vi "Axis_traversed.vi"(4 "Position array":sgl[][](array[numeric]) format="%.2f") -> (1 "Axis Traversed":enum16{"X traverse", "Y traverse", "Z traverse"}(ring))   [LabVIEW 2020]
uses:
  Globals/Trav_pos_global.vi
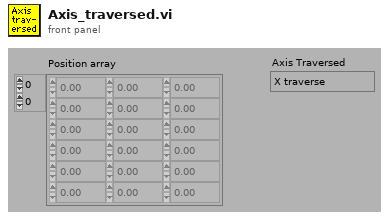
[diagram p1: front panel]
types:
  T1 = enum16{"X traverse", "Y traverse", "Z traverse"}[]
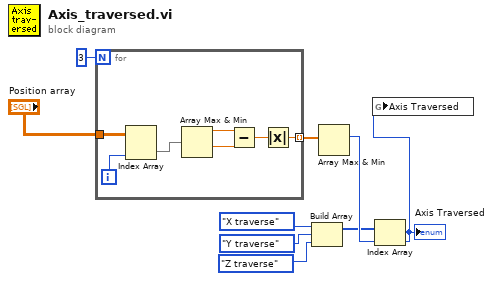
[diagram p0: block diagram]
diagram:
  n1 = for {
    N: 3 -> [_]
    tunnel: "Position array" -> [w15]
    tunnel: [w10] -> w4 mode=indexing
    i -> [w16]
    n2 = Index Array(array=w15, index (col)=w16) -> (element=w14:sgl[])  [unwired: 1 in]
    n3 = Array Max & Min(array=w14) -> (max value=w13:sgl, min value=w12:sgl)  [unwired: 2 out]
    n4 = Subtract(x=w13, y=w12) -> (x-y=w11:sgl)
    n5 = Absolute Value(x=w11) -> (abs(x)=w10:sgl)
  }
  n6 = Build Array(enum16{"X traverse", "Y traverse", "Z traverse"}."X traverse", enum16{"X traverse", "Y traverse", "Z traverse"}."Y traverse", enum16{"X traverse", "Y traverse", "Z traverse"}."Z traverse") -> (w2:T1)
  n7 = Array Max & Min(array=w4) -> (max index (indices)=w3:i32)  [unwired: 3 out]
  n8 = Index Array(array=w2, index=w3) -> (element=w1:enum16{"X traverse", "Y traverse", "Z traverse"})
  "Axis Traversed" <- w1
  n9 = global write "Trav_pos_global.vi" "Axis Traversed"(w1) -> ()
